vi "Open one tiff.vi"(1 "Pre FRAP image":path=path "F:/Andrey/Bollyky FRAP phage/pre FRAP 2_XY1729547452_Z0_T0_C0.tif") -> (0 "Frame":u16[][](array[numeric]))   [LabVIEW 2019]
uses:
  System.Drawing
  <vilib>/wsapi/NI_WebServices.lvlib
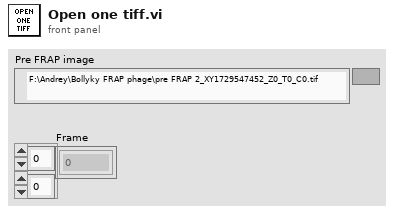
[diagram p1: front panel]
types:
  T1 = typedef "imagedata.ctl" = cluster{"image type":i32, "image depth":i32, "image":u8[], "mask":u8[], "colors":u32[], "Rectangle":cluster{"left":i16, "top":i16, "right":i16, "bottom":i16}}
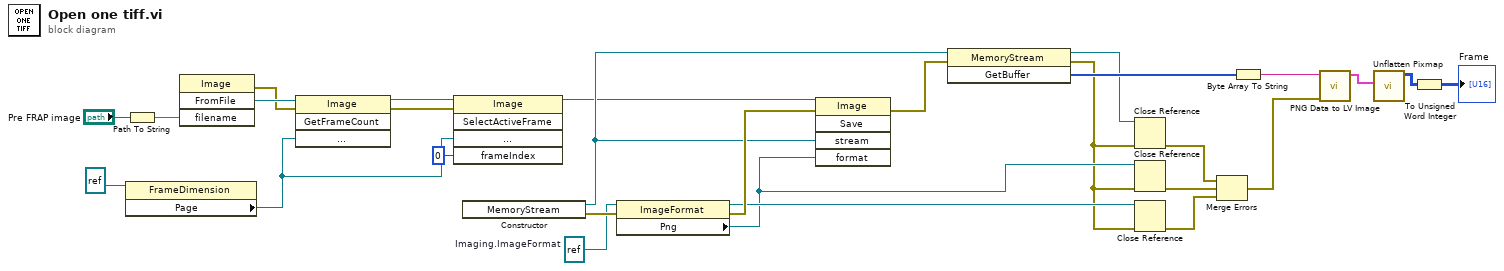
[diagram p0: block diagram]
diagram:
  w17 = refnum<k24> refnum  # Imaging.ImageFormat
  n1 = property class="FrameDimension"(reference=refnum<k24> refnum ("dimension")) -> ("Page"=w6:refnum<k24>)  [unwired: 1 in, 2 out]
  n2 = Path To String(path="Pre FRAP image") -> (string=w10:string)
  n3 = invoke class="Image" method="FromFile"("filename"=w10) -> (error out=w9:errorcluster, "FromFile"=w11:refnum<k24>)  [unwired: 3 in, 2 out]
  n4 = invoke class="Image" method="GetFrameCount"(reference=w11, error in=w9, "dimension"=w6) -> (reference out=w13:refnum<k24>, error out=w12:errorcluster)  [unwired: 1 in, 2 out]
  n5 = invoke class="Image" method="SelectActiveFrame"(reference=w13, error in=w12, "dimension"=w6, "frameIndex"=0) -> (reference out=w4:refnum<k24>)  [unwired: 1 in, 4 out]
  n6 = constructor class="MemoryStream"() -> (reference out=w15:refnum<k24>, error out=w26:errorcluster)  [unwired: 3 in, 1 out]
  n7 = property class="ImageFormat"(reference=w17, error in=w26) -> (reference out=w23:refnum<k24>, error out=w25:errorcluster, "Png"=w21:refnum<k24>)
  n8 = invoke class="Image" method="Save"(reference=w4, error in=w25, "stream"=w15, "format"=w21) -> (error out=w24:errorcluster)  [unwired: 1 in, 4 out]
  n9 = invoke class="MemoryStream" method="GetBuffer"(reference=w15, error in=w24) -> (reference out=w22:refnum<k24>, error out=w18:errorcluster, "GetBuffer"=w28:u8[])  [unwired: 1 in]
  n10 = Close Reference(reference=w22, error in (no error)=w18) -> (error out=w14:errorcluster)
  n11 = Close Reference(reference=w21, error in (no error)=w18) -> (error out=w19:errorcluster)
  n12 = Close Reference(reference=w23, error in (no error)=w18) -> (error out=w20:errorcluster)
  n13 = Merge Errors(w14, w19, w20) -> (w16:errorcluster)
  n14 = Byte Array To String(unsigned byte array=w28) -> (string=w27:string)
  n15 = call <vilib>:"PNG Data to LV Image.vi"("error in (no error)"=w16, "png data"=w27) -> ("image data"=w3:T1)  [unwired: 8 in, 1 out]
  n16 = call <vilib>:"Unflatten Pixmap.vi"("image data"=w3) -> ("24-bit pixmap"=w2:u32[][])  [unwired: 4 in, 6 out]
  n17 = To Unsigned Word Integer(number=w2) -> (unsigned 16bit integer=→"Frame":u16[][])
